vi "DWF PS Enable All Outputs.vi"(0 "Instrument Handle In":u32, 5 "Enable Outputs":bool, 11 "Error In":errorcluster caption="Error In (no error)") -> (4 "Instrument Handle Out":u32, 15 "Error Out":errorcluster)   [LabVIEW 2015, in "DigilentWF.lvlib"]
doc: "Enables or disables all outputs on all channels of the instrument."
uses:
  <vilib>/DigilentWF/DigilentWF.lvlib
  dwf.dll
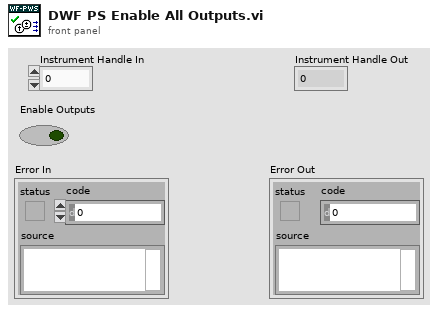
[diagram p1: front panel]
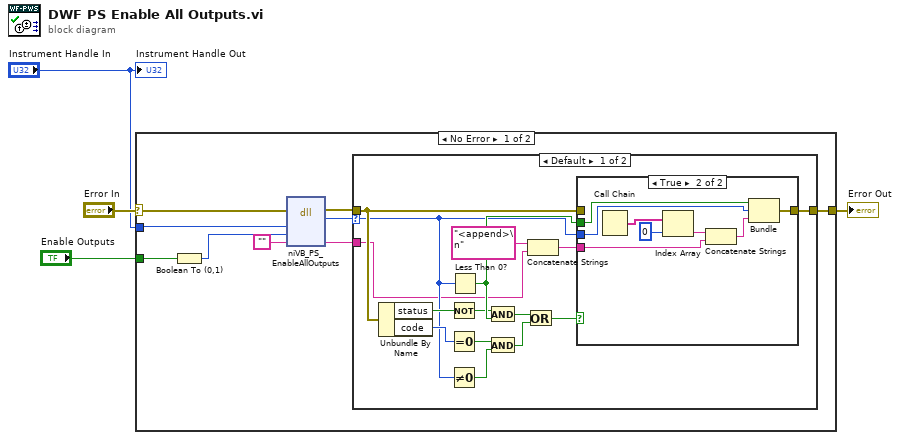
[diagram p0: block diagram]
diagram:
  n1 = case "outter_case" shown="No Error" "Error In" {
    selector: "Error In" -> [w11 w39]
    tunnel: [w13 w39] -> w3
    tunnel: "Instrument Handle In" -> [w9 _]
    tunnel: "Enable Outputs" -> [w12 _]
    frame No Error {
      n2 = Boolean To (0,1)(Boolean=w12) -> (0, 1=w8:i16)
      n3 = dll-call lib="dwf.*" fn="niVB_PS_EnableAllOutputs"(error in=w11, "instrumentHandle"=w9, "enableOutputs"=w8, "szError"="") -> (error out=w10:errorcluster, "return type"=w7:i32, "szError"=w5:string)  [unwired: 4 in, 1 out]
      n4 = case "inner_case" shown="Default" w7 {
        selector: w7 -> [w18 _]
        tunnel: w10 -> [w19 w38]
        tunnel: [w15 w38] -> w13
        tunnel: w5 -> [w14 _]
        frame Default {
          n5 = Unbundle By Name(w19) -> ("status"=w23:bool, "code"=w27:i32)
          n6 = Not(x=w23) -> (.not. x?=w26:bool)
          n7 = Equal To 0?(x=w27) -> (x = 0?=w22:bool)
          n8 = Not Equal To 0?(x=w18) -> (x != 0?=w25:bool)
          n9 = Less Than 0?(x=w18) -> (x < 0?=w28:bool)
          n10 = And(x=w26, y=w28) -> (x .and. y?=w24:bool)
          n11 = And(x=w22, y=w25) -> (x .and. y?=w21:bool)
          n12 = Or(x=w24, y=w21) -> (x .or. y?=w20:bool)
          n13 = Concatenate Strings("<append>\n" ("string"), w14) -> (w17:string)
          n14 = case shown="True" w20 {
            tunnel: [w29 w36] -> w15
            tunnel: w18 -> [_ w35]
            tunnel: w28 -> [_ w34]
            tunnel: w19 -> [w29 _]
            tunnel: w17 -> [_ w30]
            frame False {
            }
            frame True {
              n15 = Call Chain() -> (call chain=w33:string[])
              n16 = Index Array(array=w33, index=0) -> (element=w32:string)
              n17 = Concatenate Strings(w32, w30) -> (w37:string)
              n18 = Bundle(w34, "return type"=w35, w37) -> (w36:cluster{bool, "return type":i32, string})  [unwired: 1 out]
            }
          }
        }
        frame 0 {
        }
      }
    }
    frame Error {
    }
  }
  "Error Out" <- w3
  "Instrument Handle Out" <- "Instrument Handle In"
